vi "CUTUncert.vi"() -> ()   [LabVIEW 2014]
uses:
  typedefs/ePhases.ctl
  typedefs/eMainAction.ctl
  typedefs/ePathsAction.ctl
  typedefs/Alldata.ctl
  typedefs/NISTData.ctl
  typedefs/NIDataArray.ctl
  typedefs/NIData.ctl
  typedefs/PhasorRectangular.ctl
  typedefs/DUTData.ctl
  typedefs/NICalcAnalysis.ctl
  typedefs/CalcPhasorError.ctl
  typedefs/PlotDataArrays.ctl
  typedefs/PmuRawDataCluster.ctl
  typedefs/CalcAnalysis.ctl
panel:
  in  "ePhases":T1
  out "Plot":cluster{dbl, "Time":dbl, dbl[][]}(graph)
  in  "btnSave":bool
  in  "btnMultiSrcAnalysis":bool
  in  "btnExit":bool
  in  "btnSrcAnalysis":bool
  out "error out":errorcluster
  in  "error in (no error)":errorcluster
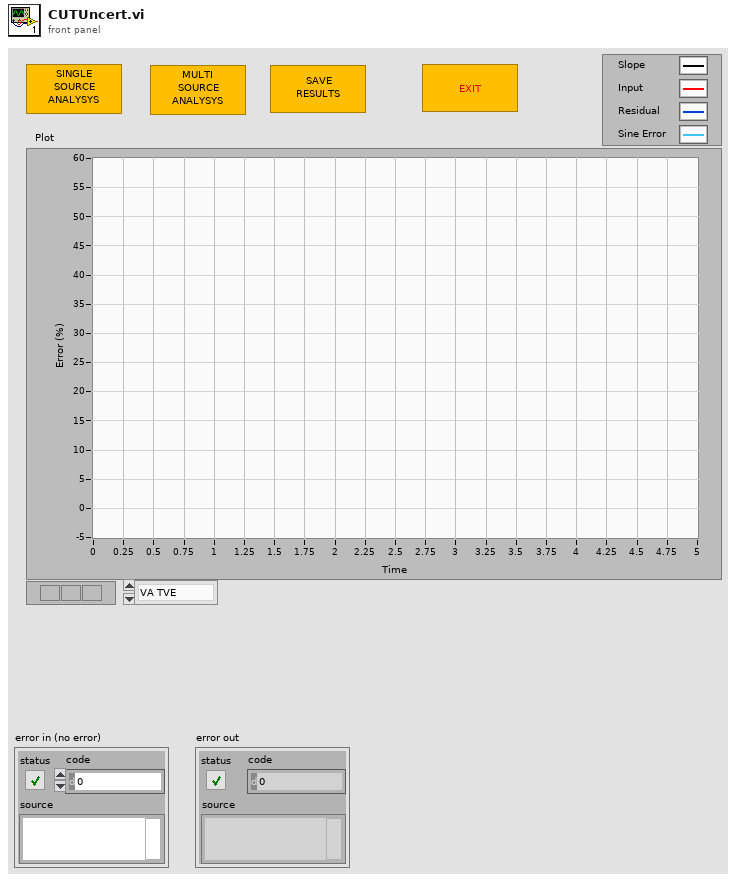
[diagram p1: front panel]
types:
  T1 = typedef "ePhases.ctl" = enum16{"VA TVE", "VA Mag ", "VA Phase", "VB TVE", "VB Mag", "VB Phase", "VC TVE", "VC Mag", "VC Phase", "V+ TVE", "V+ Mag", "V+ Phase", "IA TVE", "IA Mag", "IA Phase", "IB TVE", "IB Mag", "IB Phase", "IC TVE", "IC Mag", "IC Phase", "I+ TVE", "I+ Mag", "I+ Phase", "FE", "RFE"}
  T2 = typedef "eMainAction.ctl" = enum16{"Init", "ProcessUI", "Exit"}
  T3 = typedef "ePathsAction.ctl" = enum16{"Set", "Get", "Load", "Save", "Default", "Exit"}
  T4 = typedef "Alldata.ctl" = cluster{"NISTData":T5, "FlukeData":T12, "Params":dbl[]}
  T5 = typedef "NISTData.ctl" = cluster{"NIDataArray":T6, "DUTDataArray":T9[], "DataAnlysisArray":T10[]}
  T6 = typedef "NIDataArray.ctl" = T7[]
  T7 = typedef "NIData.ctl" = cluster{"Time":dbl, "VA":T8, "VB":T8, "VC":T8, "V+":T8, "IA":T8, "IB":T8, "IC":T8, "I+":T8, "Freq":dbl, "ROCOF":dbl, "TimeStamp":timestamp}
  T8 = typedef "PhasorRectangular.ctl" = cluster{"Real":dbl, "Imaginary":dbl}
  T9 = typedef "DUTData.ctl" = cluster{"Time":dbl, "VA":T8, "VB":T8, "VC":T8, "V1":T8, "IA":T8, "IB":T8, "IC":T8, "I1":T8, "Freq":dbl, "ROCOF":dbl, "TimeStamp":timestamp}
  T10 = typedef "NICalcAnalysis.ctl" = cluster{"Time":dbl, "VPhaseA":T11, "VPhaseB":T11, "VPhaseC":T11, "VPosSeq":T11, "IPhaseA":T11, "IPhaseB":T11, "IPhaseC":T11, "IPosSeq":T11, "Fe":dbl, "RFe":dbl, "TimeStamp":timestamp}
  T11 = typedef "CalcPhasorError.ctl" = cluster{"TVE":dbl, "MagErr":dbl, "PhaseErr":dbl}
  T12 = typedef "PlotDataArrays.ctl" = cluster{"PMUDataArray":T13[], "ModelDataArray":T13[], "DataAnalysisArray":T14[]}
  T13 = typedef "PmuRawDataCluster.ctl" = cluster{"TimeStamp":timestamp, "VPhaseA":T8, "VPhaseB":T8, "VPhaseC":T8, "VPosSeq":T8, "IPhaseA":T8, "IPhaseB":T8, "IPhaseC":T8, "IPosSeq":T8, "FREQUENCY":dbl, "ROCOF":sgl}
  T14 = typedef "CalcAnalysis.ctl" = cluster{"TimeStamp":timestamp, "VPhaseA":T11, "VPhaseB":T11, "VPhaseC":T11, "VPosSeq":T11, "IPhaseA":T11, "IPhaseB":T11, "IPhaseC":T11, "IPosSeq":T11, "Fe":dbl, "RFe":dbl}
  T15 = enum16{"VA TVE", "VA Mag ", "VA Phase", "VB TVE", "VB Mag", "VB Phase", "VC TVE", "VC Mag", "VC Phase", "V+ TVE", "V+ Mag", "V+ Phase", "IA TVE", "IA Mag", "IA Phase", "IB TVE", "IB Mag", "IB Phase", "IC TVE", "IC Mag", "IC Phase", "I+ TVE", "I+ Mag", "I+ Phase", "FE", "RFE"}
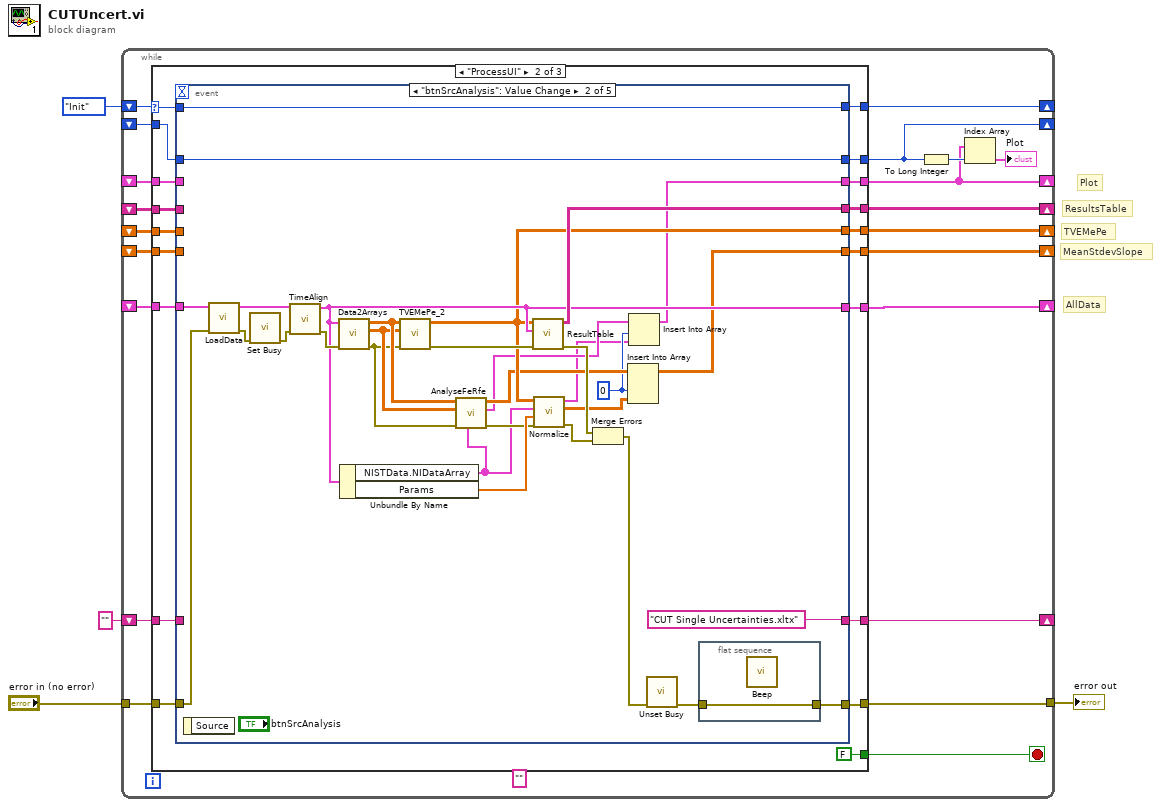
[diagram p0: block diagram]
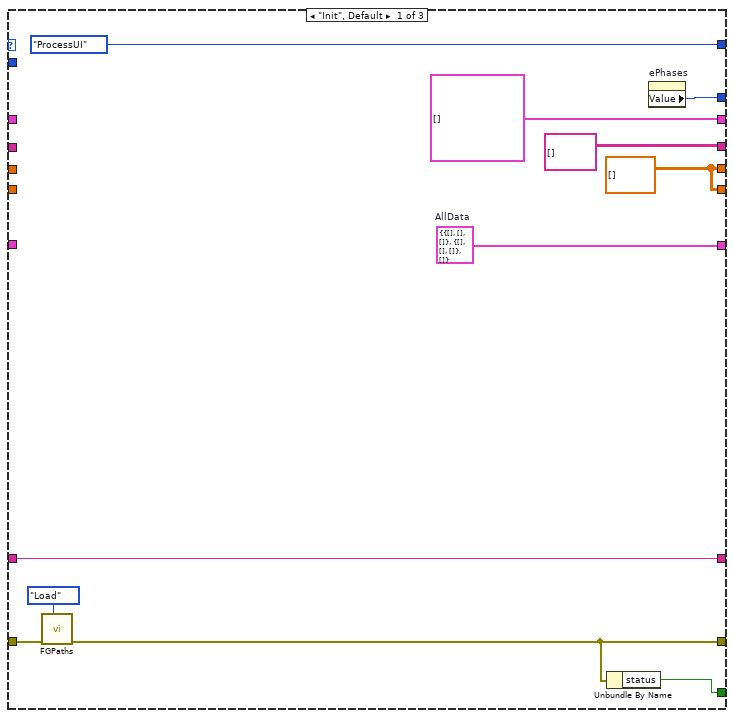
[diagram p2: hidden frame]
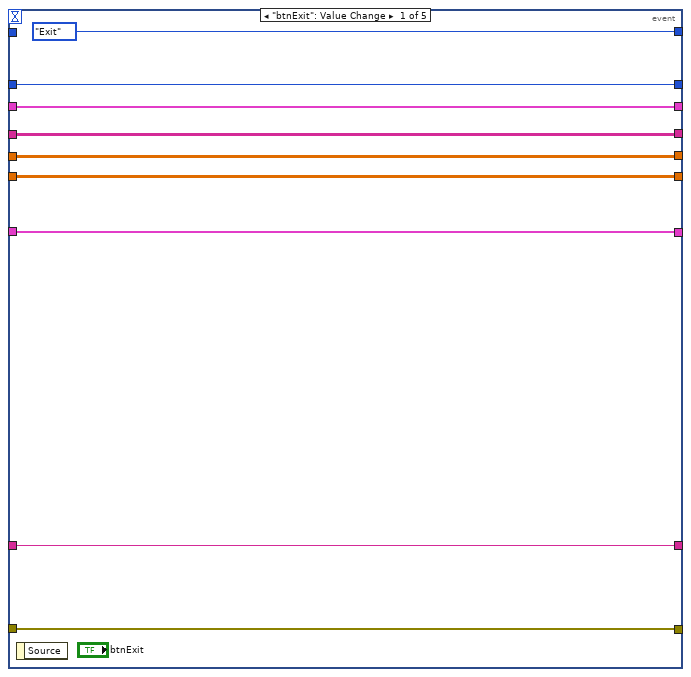
[diagram p3: hidden frame]
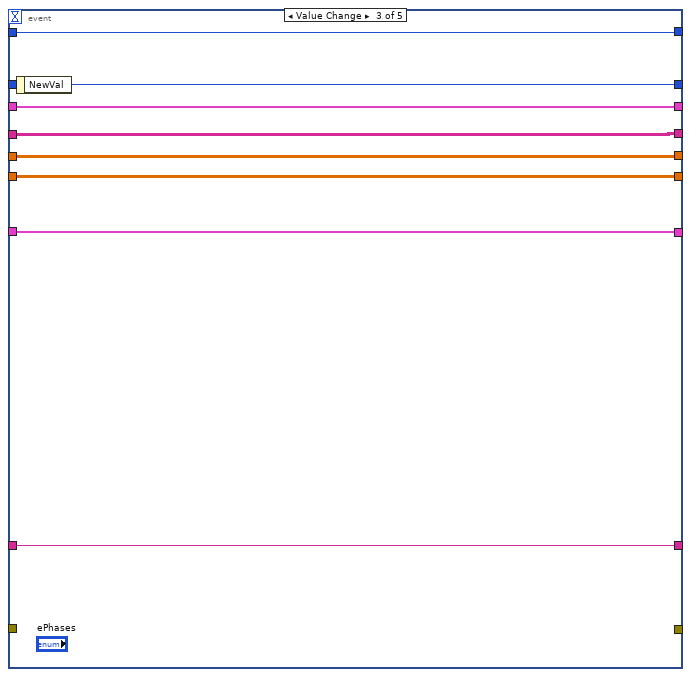
[diagram p4: hidden frame]
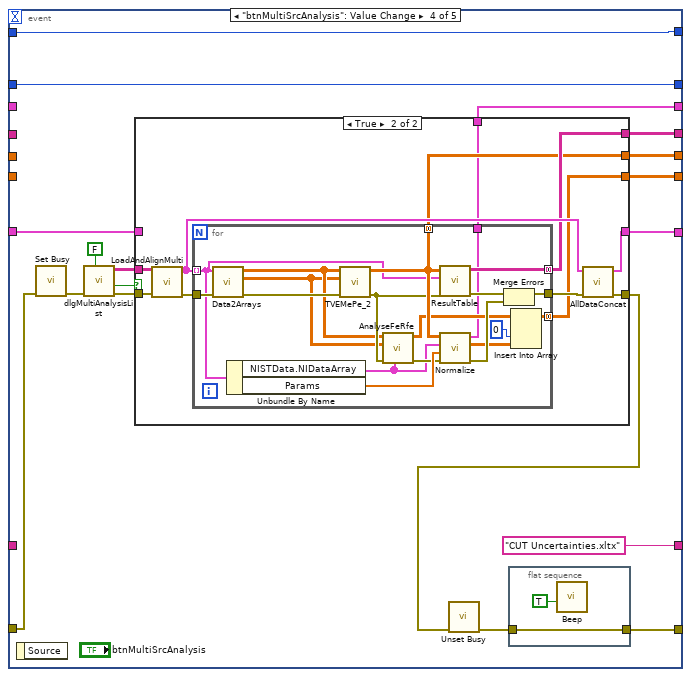
[diagram p5: hidden frame]
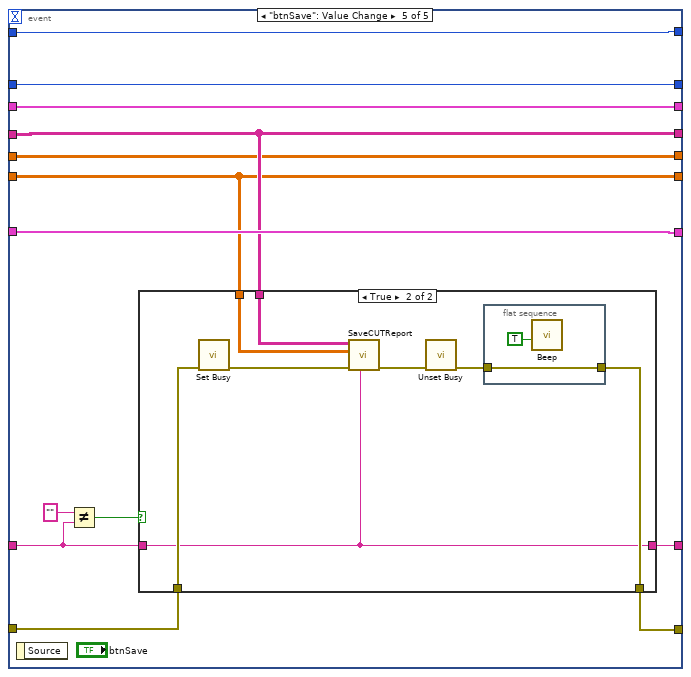
[diagram p7: hidden frame]
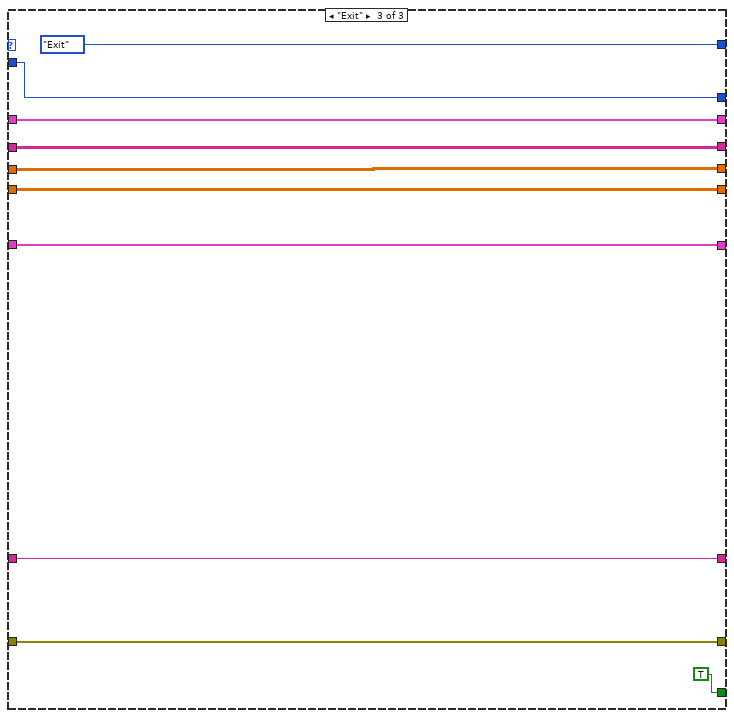
[diagram p9: hidden frame]
diagram:
  # "Plot"
  # "AllData"
  # "ResultsTable"
  # "TVEMePe"
  # "MeanStdevSlope"
  n1 = while {
    shift-right: [w23] -> _
    shift-left: eMainAction."Init" ("eMainAction") -> [w24]
    tunnel: [w22] -> w2
    tunnel: "error in (no error)" -> [w21]
    shift-right: [w19] -> _
    shift-left: _ -> [w20]
    shift-right: [w18] -> _
    shift-left: _ -> [w17]
    shift-right: [w16] -> _
    shift-left: _ -> [w15]
    shift-right: [w14] -> _
    shift-left: _ -> [w13]
    shift-right: [w12] -> _
    shift-left: "" ("TemplateName") -> [w11]
    shift-right: [w8] -> _
    shift-left: _ -> [w10]
    shift-right: [w6] -> _
    shift-left: _ -> [w5]
    stop <- w25 stop-if-true
    (unwired) ""
    n2 = case shown="\"ProcessUI\"" w24 {
      selector: w24 -> [_ w51 _]
      tunnel: [w26 FALSE TRUE] -> w25
      tunnel: [eMainAction."ProcessUI" ("eMainAction") w54 eMainAction."Exit" ("eMainAction")] -> w23
      tunnel: [w27 w52 w189] -> w22
      tunnel: w21 -> [w35 w53 w189]
      tunnel: w20 -> [_ w50 w187]
      tunnel: [w32 w49 w187] -> w19
      tunnel: [string[][] [] ("Results Table") w48 w188] -> w18
      tunnel: w17 -> [_ w47 w188]
      tunnel: [w31 w46 w186] -> w16
      tunnel: w15 -> [_ w45 w186]
      tunnel: [w31 w44 w185] -> w14
      tunnel: w13 -> [_ w43 w185]
      tunnel: [w30 w42 w184] -> w12
      tunnel: w11 -> [w30 w41 w184]
      tunnel: [cluster{dbl, "Time":dbl, dbl[][]}[] [] ("Plot Out") w40 w183] -> w8
      tunnel: w10 -> [_ w39 w183]
      tunnel: [w28 w38 w182] -> w6
      tunnel: w5 -> [_ w37 w182]
      frame "Init", Default {
        w31 = dbl[][] [] ("TVEMePe")
        w32 = T4 {"NISTData"={"NIDataArray"=[], "DUTDataArray"=[], "DataAnlysisArray"=[]}, "FlukeData"={"PMUDataArray"=[], "ModelDataArray"=[], "DataAnalysisArray"=[]}, "Params"=[]}  # AllData
        n3 = call "FGPaths.vi"("ePathsAction"=ePathsAction."Load", "error in (no error)"=w35) -> ("error out"=w27:errorcluster)  [unwired: 8 in, 1 out]
        n4 = Unbundle By Name(w27) -> ("status"=w26:bool)
        n5 = property on="ePhases" class="Enum (strict)"() -> ("Value"=w28:T15)  [unwired: 2 in, 2 out]
      }
      frame "ProcessUI" {
        n6 = event shown="[1] \"btnSrcAnalysis\": Value Change" {
          selector: _ -> [_ _ _ _ _]
          dyn-events: _ -> [_ _ _ _ _]
          timeout: _ -> [_ _ _ _ _]
          tunnel: [eMainAction."Exit" ("eMainAction") w95 w97 w115 w169] -> w54
          tunnel: [w63 w85 _ w108 w163] -> w52
          tunnel: w53 -> [w63 w94 _ w122 w167]
          tunnel: w51 -> [_ w95 w97 w115 w169]
          tunnel: w50 -> [w61 w93 w102 w116 w168]
          tunnel: [w61 w83 w102 w114 w168] -> w49
          tunnel: [w62 w87 w99 w113 w166] -> w48
          tunnel: w47 -> [w62 _ w99 _ w166]
          tunnel: [w60 w75 w100 w112 w165] -> w46
          tunnel: w45 -> [w60 _ w100 _ w165]
          tunnel: [w59 w69 w101 w111 w164] -> w44
          tunnel: w43 -> [w59 _ w101 _ w164]
          tunnel: [w58 "CUT Single Uncertainties.xltx" ("TemplateName") w103 "CUT Uncertainties.xltx" ("TemplateName") w159] -> w42
          tunnel: w41 -> [w58 _ w103 _ w162]
          tunnel: [w57 w65 w98 w106 w158] -> w40
          tunnel: w39 -> [w57 _ w98 _ w158]
          tunnel: [w56 w70 w104 w105 w157] -> w38
          tunnel: w37 -> [w56 w70 _ w105 w157]
          event "btnExit": Value Change {
            n7 = event-data() -> ()  [unwired: 1 in, 1 out]
          }
          event "btnSrcAnalysis": Value Change {
            w67 = 0 ("index (row)")
            n8 = event-data() -> ()  [unwired: 1 in, 1 out]
            n9 = call "LoadData.vi"("error in (no error)"=w94, "AllData In"=w93) -> ("error out"=w92:errorcluster, "AllData Out"=w91:T4)  [unwired: 8 in]
            n10 = call <vilib>:"Set Busy.vi"("error in (no error)"=w92) -> ("error out"=w90:errorcluster)  [unwired: 9 in, 1 out]
            n11 = call "TimeAlign.vi"("error in (no error)"=w90, "AllData In"=w91) -> ("error out"=w89:errorcluster, "AllData Out"=w83:T4)  [unwired: 8 in]
            n12 = call "Data2Arrays.vi"("error in (no error)"=w89, "AllData"=w83) -> ("error out"=w80:errorcluster, "Fluke"=w81:dbl[][], "NIST"=w82:dbl[][])  [unwired: 7 in]
            n13 = Unbundle By Name(w83) -> ("NISTData.NIDataArray"=w73:T6, "Params"=w84:dbl[])
            n14 = call "TVEMePe_2.vi"("error in (no error)"=w80, "Fluke"=w81, "NIST"=w82) -> ("error out"=w88:errorcluster, "TVEMePe"=w75:dbl[][])  [unwired: 7 in]
            n15 = call "AnalyseFeRfe.vi"("NISTData.NIDataArray"=w73, "error in (no error)"=w80, "Fluke"=w81, "NIST"=w82) -> ("error out"=w79:errorcluster, "Plot"=w68:cluster{dbl, "Time":dbl, dbl[][]}[], "FERfe Stats"=w74:dbl[][])  [unwired: 5 in]
            n16 = call "ResultTable.vi"("error in (no error)"=w88, "AllData"=w83, "TVEMePe"=w75) -> ("error out"=w77:errorcluster, "Results Table"=w87:string[][])  [unwired: 7 in]
            n17 = call "Normalize.vi"("error in (no error)"=w79, "Params"=w84, "NISTData.NIDataArray"=w73, "TVEMePe"=w75) -> ("error out"=w78:errorcluster, "MeanStdevSlopeSineAmpl"=w72:dbl[][], "Plot Out"=w66:cluster{dbl, "Time":dbl, dbl[][]}[])  [unwired: 4 in, 1 out]
            n18 = Merge Errors(w77, w78) -> (w76:errorcluster)
            n19 = Insert Into Array(array=w74, index (col)=w67, new element=w72) -> (w69:dbl[][])  [unwired: 1 in]
            n20 = Insert Into Array(array=w68, index=w67, new element=w66) -> (w65:cluster{dbl, "Time":dbl, dbl[][]}[])
            n21 = call <vilib>:"Unset Busy.vi"("error in (no error)"=w76) -> ("error out"=w86:errorcluster)  [unwired: 10 in]
            n22 = flat-sequence {
              tunnel: [w96] -> w85
              tunnel: w86 -> [w96]
              frame #0 {
                n23 = call <vilib>:"Beep.vi"() -> ()  [unwired: 12 in]
              }
            }
          }
          event Value Change {
            n24 = event-data() -> ("NewVal"=w104:T1)  [unwired: 1 in]
          }
          event "btnMultiSrcAnalysis": Value Change {
            n25 = event-data() -> ()  [unwired: 1 in, 1 out]
            n26 = call <vilib>:"Set Busy.vi"("error in (no error)"=w122) -> ("error out"=w121:errorcluster)  [unwired: 9 in, 1 out]
            n27 = call "dlgMultiAnalysisList.vi"("StandAlone (true)"=FALSE, "error in (no error)"=w121) -> ("error out"=w118:errorcluster, "Analyse"=w119:bool, "FileList"=w117:string[][])  [unwired: 7 in]
            n28 = case shown="True" w119 {
              tunnel: w118 -> [w125 w137]
              tunnel: w117 -> [_ w136]
              tunnel: [w126 w135] -> w114
              tunnel: w116 -> [w126 _]
              tunnel: [w125 w134] -> w110
              tunnel: [_ w130] -> w113
              tunnel: [_ w129] -> w112
              tunnel: [_ w128] -> w111
              tunnel: [_ w127] -> w106
              frame False {
              }
              frame True {
                n29 = call "LoadAndAlignMulti.vi"("error in (no error)"=w137, "FileList"=w136) -> ("error out"=w133:errorcluster, "AllDataArray"=w132:T4[])  [unwired: 8 in]
                n30 = for {
                  tunnel: w132 -> [w150] mode=indexing
                  tunnel: w133 -> [w156]
                  tunnel: [w149] -> w131
                  tunnel: [w152] -> w130 mode=concatenating
                  tunnel: [w151] -> w129 mode=concatenating
                  tunnel: [w140] -> w128 mode=concatenating
                  tunnel: [w138] -> w127
                  n31 = call "Data2Arrays.vi"("error in (no error)"=w156, "AllData"=w150) -> ("error out"=w154:errorcluster, "Fluke"=w143:dbl[][], "NIST"=w144:dbl[][])  [unwired: 7 in]
                  n32 = Unbundle By Name(w150) -> ("NISTData.NIDataArray"=w145:T6, "Params"=w155:dbl[])
                  n33 = call "TVEMePe_2.vi"("error in (no error)"=w154, "Fluke"=w143, "NIST"=w144) -> ("error out"=w147:errorcluster, "TVEMePe"=w151:dbl[][])  [unwired: 7 in]
                  n34 = call "AnalyseFeRfe.vi"("NISTData.NIDataArray"=w145, "error in (no error)"=w147, "Fluke"=w143, "NIST"=w144) -> ("error out"=w146:errorcluster, "FERfe Stats"=w141:dbl[][])  [unwired: 5 in, 1 out]
                  n35 = call "ResultTable.vi"("error in (no error)"=w147, "AllData"=w150, "TVEMePe"=w151) -> ("error out"=w153:errorcluster, "Results Table"=w152:string[][])  [unwired: 7 in]
                  n36 = call "Normalize.vi"("error in (no error)"=w146, "Params"=w155, "NISTData.NIDataArray"=w145, "TVEMePe"=w151) -> ("error out"=w148:errorcluster, "MeanStdevSlopeSineAmpl"=w142:dbl[][], "Plot Out"=w138:cluster{dbl, "Time":dbl, dbl[][]}[])  [unwired: 4 in, 1 out]
                  n37 = Merge Errors(w153, w148) -> (w149:errorcluster)
                  n38 = Insert Into Array(array=w141, index (col)=0 ("disabled index (col)"), new element=w142) -> (w140:dbl[][])  [unwired: 1 in]
                }
                n39 = call "AllDataConcat.vi"("error in (no error)"=w131, "AllDataArray"=w132) -> ("error out"=w134:errorcluster, "AllData"=w135:T4)  [unwired: 8 in]
              }
            }
            n40 = call <vilib>:"Unset Busy.vi"("error in (no error)"=w110) -> ("error out"=w109:errorcluster)  [unwired: 10 in]
            n41 = flat-sequence {
              tunnel: [w124] -> w108
              tunnel: w109 -> [w124]
              frame #0 {
                n42 = call <vilib>:"Beep.vi"("use system alert? (T)"=TRUE) -> ()  [unwired: 11 in]
              }
            }
          }
          event "btnSave": Value Change {
            n43 = event-data() -> ()  [unwired: 1 in, 1 out]
            n44 = Not Equal?(x="", y=w162) -> (x != y?=w160:bool)
            n45 = case shown="True" w160 {
              tunnel: w167 -> [w171 w179]
              tunnel: w166 -> [_ w177]
              tunnel: w164 -> [_ w176]
              tunnel: [w171 w173] -> w163
              tunnel: w162 -> [w170 w172]
              tunnel: [w170 w172] -> w159
              frame False {
              }
              frame True {
                n46 = call <vilib>:"Set Busy.vi"("error in (no error)"=w179) -> ("error out"=w175:errorcluster)  [unwired: 9 in, 1 out]
                n47 = call "SaveCUTReport.vi"("TemplateName"=w172, "error in (no error)"=w175, "MeanStdSlope"=w176, "Results Table"=w177) -> ("error out"=w178:errorcluster)  [unwired: 7 in]
                n48 = call <vilib>:"Unset Busy.vi"("error in (no error)"=w178) -> ("error out"=w174:errorcluster)  [unwired: 10 in]
                n49 = flat-sequence {
                  tunnel: [w181] -> w173
                  tunnel: w174 -> [w181]
                  frame #0 {
                    n50 = call <vilib>:"Beep.vi"("use system alert? (T)"=TRUE) -> ()  [unwired: 11 in]
                  }
                }
              }
            }
          }
        }
      }
      frame "Exit" {
      }
    }
    n51 = To Long Integer(number=w6) -> (32bit integer=w9:i32)
    n52 = Index Array(array=w8, index=w9) -> (element=→"Plot":cluster{dbl, "Time":dbl, dbl[][]})
  }
  "error out" <- w2
